vi "DatToIni.vi"(8 "error in (no error)":errorcluster, 11 "UserManagement in":refnum<class "UserManagement.lvclass">) -> (0 "error out":errorcluster, 3 "UserManagement out":refnum<class "UserManagement.lvclass">)   [LabVIEW 2019, in "UserManagement.lvlib" / "UserManagement.lvclass"]
uses:
  UserManagement.lvclass
  UserManagement.lvclass/UserManagement.ctl
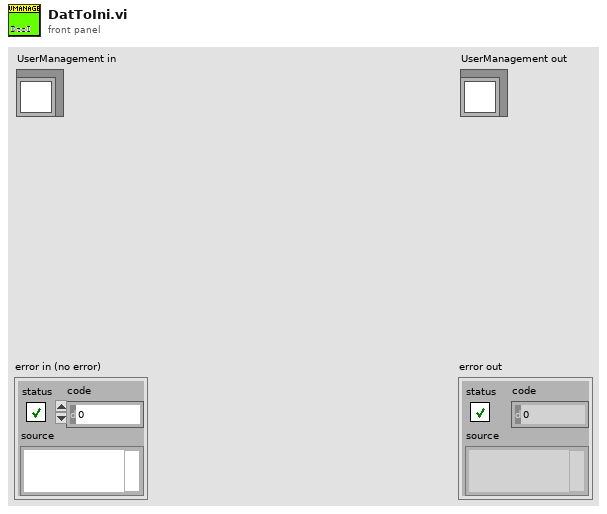
[diagram p1: front panel]
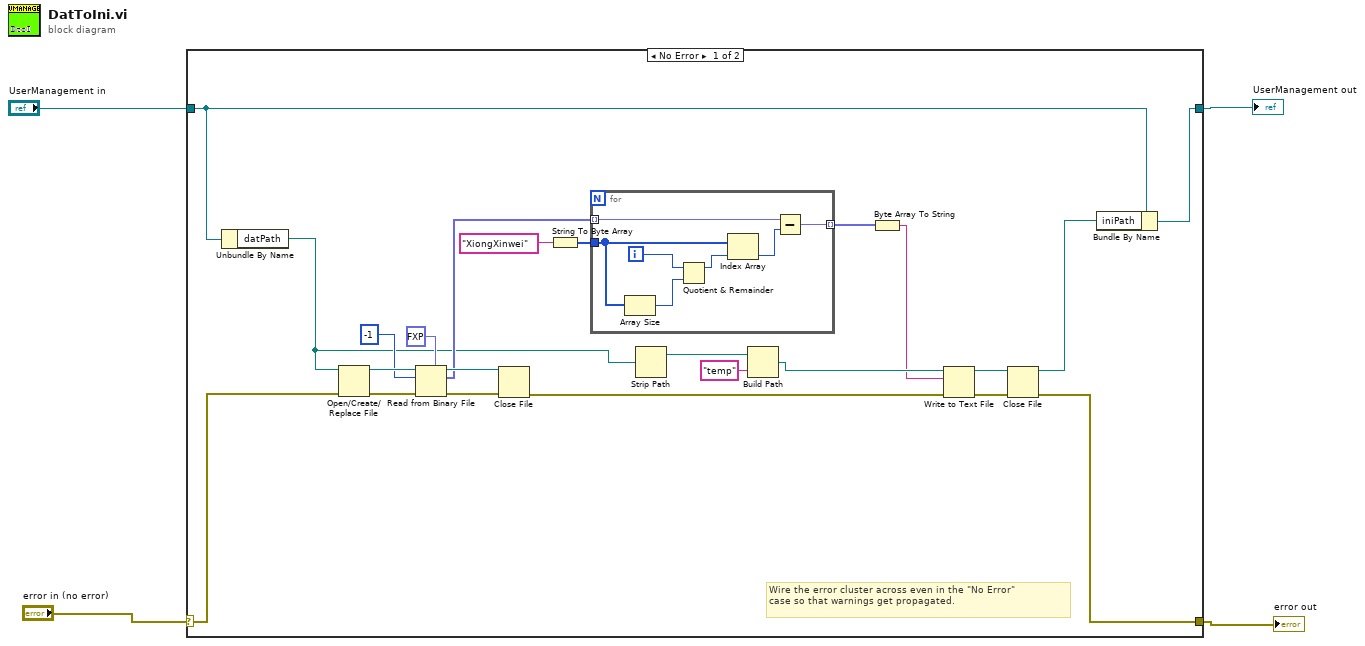
[diagram p0: block diagram]
diagram:
  n1 = case shown="No Error" "error in (no error)" {
    selector: "error in (no error)" -> [w9 w36]
    tunnel: [w5 w36] -> w1
    tunnel: [w6 w35] -> w2
    tunnel: "UserManagement in" -> [w8 w35]
    frame No Error {
      # "Wire the error cluster across even in the \"No Error\"\ncase so that warnings get propagated."
      n2 = Unbundle By Name(w8) -> ("datPath"=w10:path)
      n3 = Open/Create/Replace File(file path (use dialog)=w10, error in=w9) -> (refnum out=w27:refnum<file>, error out=w26:errorcluster)  [unwired: 4 in, 1 out]
      n4 = Read from Binary File(5:fxp<+,8,8> 0.0 ("总数(1)"), 8:w26, 10:-1 ("总数(1)"), 11:w27) -> (0:w23:errorcluster, 2:w21:fxp<+,8,8>[], 3:w24:refnum<file>)  [unwired: 2 in, 1 out]
      n5 = Close File(refnum=w24, error in=w23) -> (error out=w17:errorcluster)  [unwired: 1 out]
      n6 = String To Byte Array(string="XiongXinwei" ("字符串")) -> (unsigned byte array=w19:u8[])
      n7 = for {
        tunnel: w21 -> [w30] mode=indexing
        tunnel: w19 -> [w31]
        tunnel: [w28] -> w18 mode=indexing
        i -> [w33]
        n8 = Array Size(array=w31) -> (size(s)=w34:i32)
        n9 = Quotient & Remainder(x=w33, y=w34) -> (x-y*floor(x/y)=w32:i32)  [unwired: 1 out]
        n10 = Index Array(array=w31, index=w32) -> (element=w29:u8)
        n11 = Subtract ("减")(x=w30, y=w29) -> (x-y=w28:fxp<+,8,8>)
      }
      n12 = Strip Path(path=w10) -> (stripped path=w16:path)  [unwired: 1 out]
      n13 = Build Path(base path=w16, name or relative path="temp" ("名称或相对路径")) -> (appended path=w14:path)
      n14 = Byte Array To String(unsigned byte array=w18) -> (string=w13:string)
      n15 = Write to Text File(file (use dialog)=w14, text=w13, error in=w17) -> (refnum out=w12:refnum<file>, error out=w11:errorcluster)  [unwired: 1 in, 1 out]
      n16 = Close File(refnum=w12, error in=w11) -> (path=w7:path, error out=w5:errorcluster)
      n17 = Bundle By Name(cluster=w8, "iniPath"=w7) -> (w6:refnum<class "UserManagement.lvclass">)
    }
    frame Error {
    }
  }
  "error out" <- w1
  "UserManagement out" <- w2
